vi "Robot Global Data.vi"() -> ()   [LabVIEW 2012]
doc: "This global VI can contain as many global variables as you need. Place a control on the panel, give it a good name. To read or write to it from a VI, drag the icon to the diagram of that VI. You can also drag from the project. Click on the node to change which global you access. You shouldn't have multiple locations writing to a global or it will cause a race-condition."
uses:
  <vilib>/Rock Robotics/WPI/Camera/WPI_CameraImageSize.ctl
  <vilib>/Rock Robotics/WPI/DriverStation/WPI_DriverStationRobotMode2.ctl
panel:
  in  "cPresetPyramid":bool
  in  "cPresetShort":bool
  in  "cPresetMid":bool
  in  "cPresetFar":bool
  in  "cLauncherWheel":bool
  in  "cFirePneumatic":bool
  in  "cRpmControl":dbl(slide) step=0.2 scale=-1.0..1.0 scale format="%#_3g"
  in  "cAngleControl":dbl(slide) step=0.2 scale=-1.0..1.0 scale format="%#_3g"
  in  "cHalfSpeed":bool
  in  "sGyro":dbl
  in  "ControlOverride":bool
  in  "cTankDriveRight":dbl(slide) step=0.2 scale=-1.0..1.0 scale format="%#_3g"
  in  "cTankDriveLeft":dbl(slide) step=0.2 scale=-1.0..1.0 scale format="%#_3g"
  in  "Robot Mode":T1
  in  "LED toggle rate (ms)":u32=20
  in  "image size":T2
  in  "Enable Vision":bool
  # "DRIVER"
  # "SHOOTER"
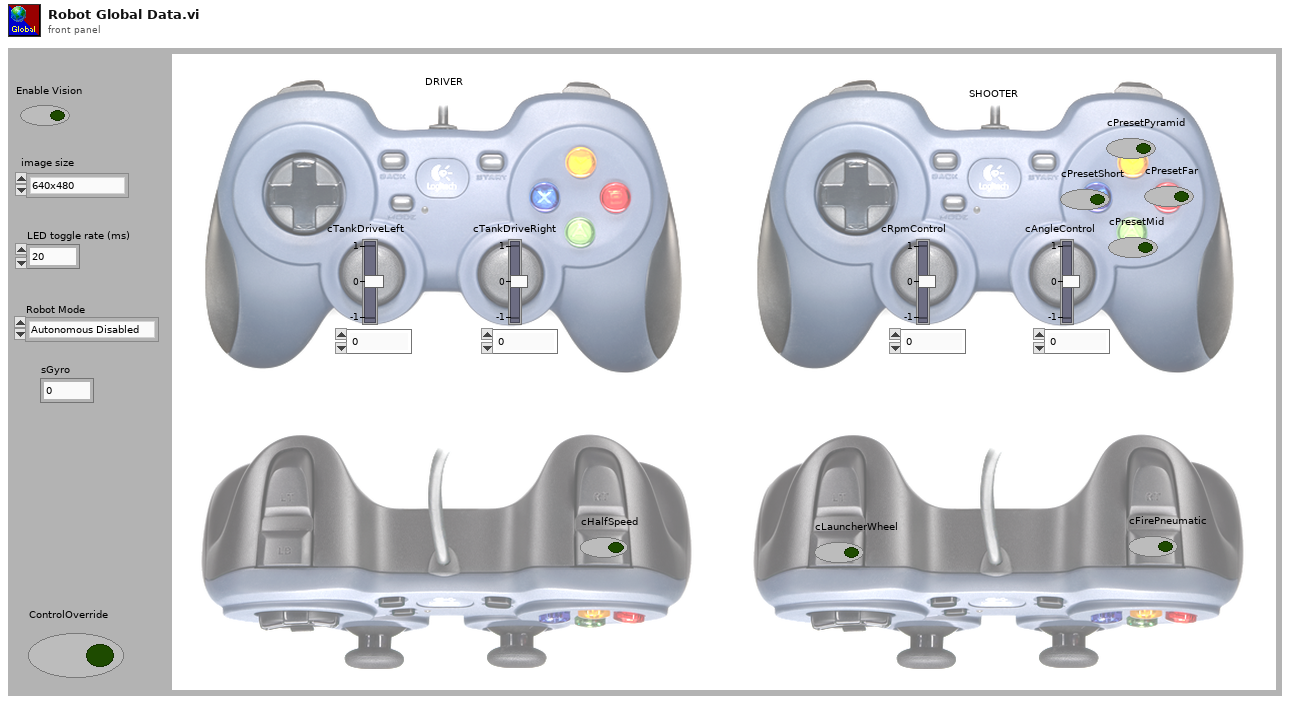
[diagram p1: front panel]
types:
  T1 = typedef "WPI_DriverStationRobotMode2.ctl" = enum16{"Autonomous Disabled", "Autonomous Enabled", "Teleop Disabled", "Teleop Enabled", "Timeout", "Finish", "Test Disabled", "Test Enabled"}
  T2 = typedef "WPI_CameraImageSize.ctl" = enum16{"640x480", "320x240", "160x120"}
diagram:
